vi "member_data_save.vi"(0 "NOC":i32, 1 "Username":string) -> ()   [LabVIEW 2014]
uses:
  <vilib>/Utility/file.llb/Read From Spreadsheet File (string).vi
  <vilib>/Utility/file.llb/Write To Spreadsheet File (string).vi
panel:
  out "all rows 2":string[][](array[string])=[["AA", "BB", "2"], ["BB", "CC", "25"]]
  out "all rows":string[][](array[string])=[["AA", "BB", "0"], ["BB", "CC", "25"]]
  out "file path":path
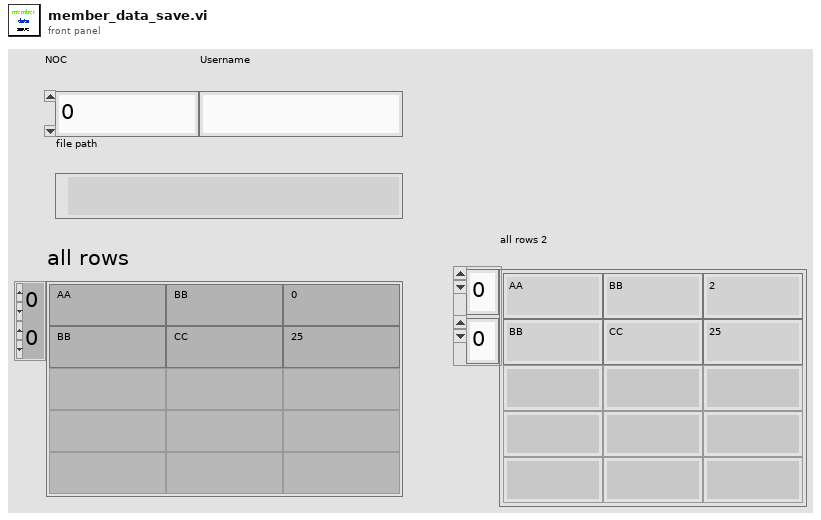
[diagram p1: front panel]
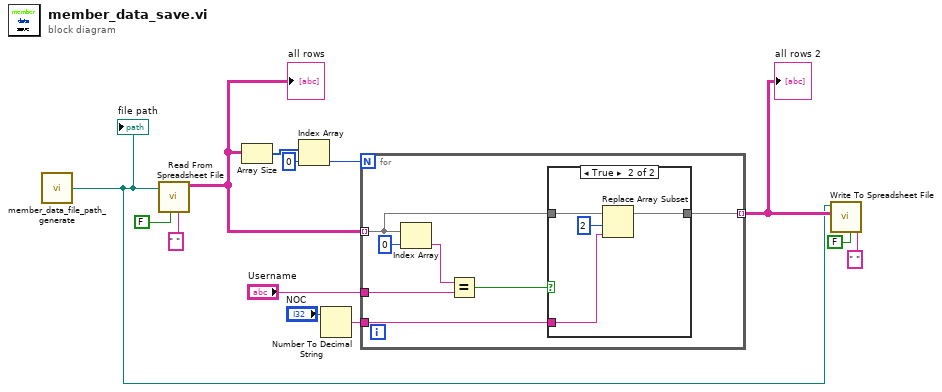
[diagram p0: block diagram]
diagram:
  n1 = call "member_data_file_path_generate.vi"() -> ("appended path"=w1:path)
  "file path" <- w1
  n2 = call-poly <vilib>:"Read From Spreadsheet File.vi"("delimiter (\\t)"=" " ("delimiter (\\t)"), "transpose (no:F)"=FALSE, "file path (dialog if empty)"=w1) -> ("all rows"=w7:string[][])  [unwired: 4 in, 4 out]
  "all rows" <- w7
  n3 = Array Size(array=w7) -> (size(s)=w10:i32[])
  n4 = Index Array(array=w10, index=0) -> (element=w8:i32)
  n5 = Number To Decimal String(number="NOC") -> (decimal integer string=w5:string)  [unwired: 1 in]
  n6 = for {
    N: w8 -> [_]
    tunnel: w7 -> [w16] mode=indexing
    tunnel: "Username" -> [w18]
    tunnel: w5 -> [w15]
    tunnel: [w14] -> w4 mode=indexing
    n7 = Index Array(array=w16, index=0) -> (element=w19:string)
    n8 = Equal?(x=w19, y=w18) -> (x = y?=w17:bool)
    n9 = case shown="True" w17 {
      tunnel: w16 -> [w21 w25]
      tunnel: w15 -> [_ w24]
      tunnel: [w21 w22] -> w14
      frame False {
      }
      frame True {
        n10 = Replace Array Subset(array=w25, new element=w24, index=2) -> (w22:string[])
      }
    }
  }
  "all rows 2" <- w4
  n11 = call-poly <vilib>:"Write To Spreadsheet File.vi"("delimiter (\\t)"=" " ("delimiter (\\t)"), "transpose? (no:F)"=FALSE, "2D data"=w4, "file path (dialog if empty)"=w1) -> ()  [unwired: 4 in, 1 out]
